vi "AMZ_S3_ERR_Check Error and Get Call Result.vi"(8 "error in (no error)":errorcluster, 10 "Response body":string, 11 "Response header":string) -> (0 "error out":errorcluster, 1 "Call Result":T1, 2 "Response body dup":string, 3 "Response header dup":string, 4 "Redirect endpoint":string, 5 "500 Or Throttled?":bool=TRUE)   [LabVIEW 2015, in "LV Interface for Amazon S3.lvlib"]
doc: "Check the respnse header and body if necessary to obtain the call's result (Success or Error codes)."
uses:
  LV Interface for Amazon S3.lvlib
  Typedefs/AMZ_S3_Call Results.ctl
  XML Parser/XML Parser.lvlib
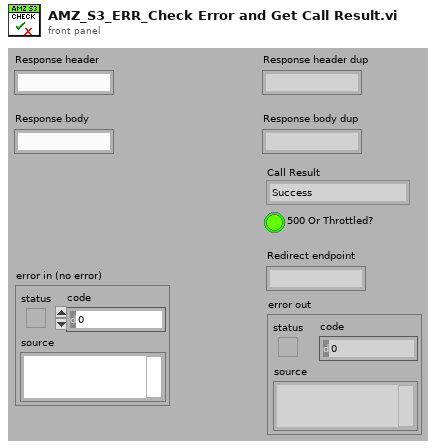
[diagram p1: front panel]
types:
  T1 = typedef "LV Interface for Amazon S3.lvlib/AMZ_S3_Call Results.ctl" = enum16{"Success", "UndefinedError", "AccessDenied", "AccountProblem", "AmbiguousGrantByEmailAddress", "BadDigest", "BucketAlreadyExists", "BucketAlreadyOwnedByYou", "BucketNotEmpty", "CredentialsNotSupported", "CrossLocationLoggingProhibited", "EntityTooSmall", "EntityTooLarge", "ExpiredToken", "IllegalVersioningConfigurationException", "IncompleteBody", "IncorrectNumberOfFilesInPostRequest", "InlineDataTooLarge", "InternalError", "InvalidAccessKeyId", "InvalidAddressingHeader", "InvalidArgument", "InvalidBucketName", "InvalidDigest", "InvalidLocationConstraint", "InvalidPart", "InvalidPartOrder", "InvalidPayer", "InvalidPolicyDocument", "InvalidRange", "InvalidSecurity", "InvalidSOAPRequest", "InvalidStorageClass", "InvalidTargetBucketForLogging", "InvalidToken", "InvalidURI", "KeyTooLong", "MalformedACLError", "MalformedPOSTRequest", "MalformedXML", "MaxMessageLengthExceeded", "MaxPostPreDataLengthExceededError", "MetadataTooLarge", "MethodNotAllowed", "MissingAttachment", "MissingContentLength", "MissingRequestBodyError", "MissingSecurityElement", "MissingSecurityHeader", "NoLoggingStatusForKey", "NoSuchBucket", "NoSuchKey", "NoSuchUpload", "NoSuchVersion", "NotImplemented", "NotSignedUp", "OperationAborted", "PermanentRedirect", "PreconditionFailed", "Redirect", "RequestIsNotMultiPartContent", "RequestTimeout", "RequestTimeTooSkewed", "RequestTorrentOfBucketError", "SignatureDoesNotMatch", "SlowDown", "TemporaryRedirect", "TokenRefreshRequired", "TooManyBuckets", "UnexpectedContent", "UnresolvableGrantByEmailAddress", "UserKeyMustBeSpecified", "LabVIEWError"}
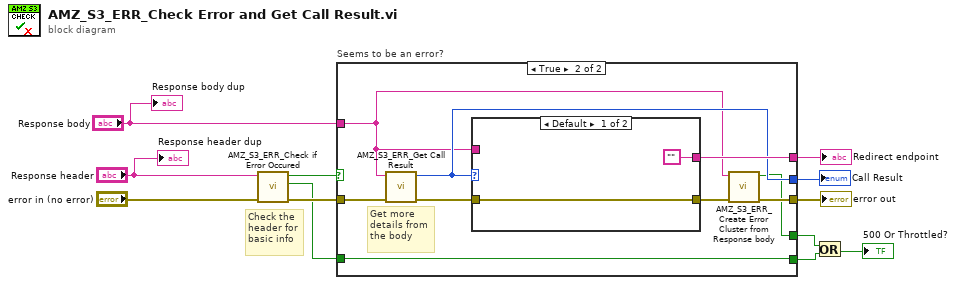
[diagram p0: block diagram]
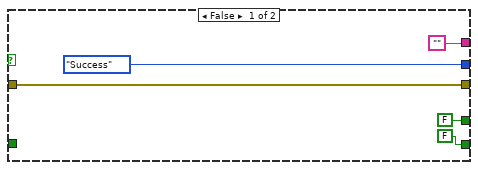
[diagram p2: hidden frame]
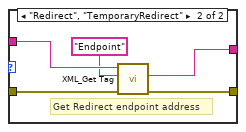
[diagram p3: hidden frame]
diagram:
  # "Check the\nheader for\nbasic info"
  n1 = call "AMZ_S3_ERR_Check if Error Occured.vi"("error in (no error)"="error in (no error)", "Response header"="Response header") -> ("error out"=w9:errorcluster, "500 Error?"=w4:bool, "Error Occured?"=w10:bool)  [unwired: 7 in]
  n2 = case "Seems to be an error?" shown="True" w10 {
    tunnel: w9 -> [w17 w26]
    tunnel: "Response body" -> [_ w20]
    tunnel: [w17 w21] -> w6
    tunnel: [AMZ_S3_Call_Results."Success" ("Call Result") w24] -> w7
    tunnel: ["" w25] -> w5
    tunnel: [FALSE ("Is Redirect?") w19] -> w1
    tunnel: [FALSE ("500 Error?") w18] -> w3
    tunnel: w4 -> [_ w18]
    frame False {
    }
    frame True {
      # "Get more\ndetails from\nthe body"
      n3 = call "AMZ_S3_ERR_Get Call Result.vi"("error in (no error)"=w26, "Response body"=w20) -> ("error out"=w23:errorcluster, "Call Result"=w24:T1)  [unwired: 8 in]
      n4 = case shown="Default" w24 {
        tunnel: w20 -> [_ w33]
        tunnel: ["" w31] -> w25
        tunnel: [w27 w30] -> w22
        tunnel: w23 -> [w27 w29]
        frame Default {
        }
        frame "Redirect", "TemporaryRedirect" {
          # "Get Redirect endpoint address"
          n5 = call "XML_Get Tag.vi"("error in (no error)"=w29, "Tag name"="Endpoint", "XML String in"=w33) -> ("error out"=w30:errorcluster, "Tag value"=w31:string)  [unwired: 4 in, 3 out]
        }
      }
      n6 = call "AMZ_S3_ERR_Create Error Cluster from Response body.vi"("error in (no error)"=w22, "Response body"=w20) -> ("error out"=w21:errorcluster, "Is Redirect?"=w19:bool)  [unwired: 8 in]
    }
  }
  "Call Result" <- w7
  "error out" <- w6
  "Redirect endpoint" <- w5
  n7 = Or(x=w1, y=w3) -> (x .or. y?=→"500 Or Throttled?":bool)
  "Response header dup" <- "Response header"
  "Response body dup" <- "Response body"
